vi "MakeWorkFile.vi"(5 "ExpFilePath":path=path "C:/Data/Matias/NewSoft_test/201707071638.h5") -> (2 "WorkFilePath":path)   [LabVIEW 2013]
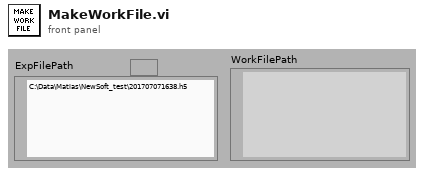
[diagram p1: front panel]
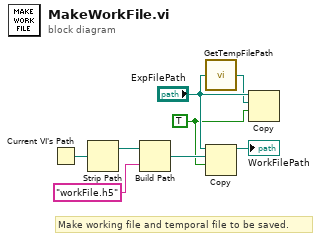
[diagram p0: block diagram]
diagram:
  w2 = TRUE
  # "Make working file and temporal file to be saved."
  n1 = Current VI's Path() -> (path=w5:path)
  n2 = Strip Path(path=w5) -> (stripped path=w4:path)  [unwired: 1 out]
  n3 = Build Path(base path=w4, name or relative path="workFile.h5") -> (appended path=w7:path)
  n4 = call "GetTempFilePath.vi"("ExpFilePath"="ExpFilePath") -> ("Temp file path"=w1:path)
  n5 = Copy(9:w2, 10:w7, 11:"ExpFilePath") -> (3:→"WorkFilePath":path)  [unwired: 2 in, 2 out]
  n6 = Copy(9:w2, 10:w1, 11:"ExpFilePath") -> ()  [unwired: 2 in, 3 out]
